vi "power calculations.vi"() -> ()   [LabVIEW 2012]
uses:
  <vilib>/measure/maspectr.llb/FFT Power Spectrum and PSD for 1 Chan.vi
  <instrlib>/niUSRP/niUSRP Fetch Rx Data (CDB Cluster).vi
  <vilib>/measure/NI_MAPro.lvlib
panel:
  in  "carrier frequency":dbl=100000.0 format="%#_6p"
  in  "gain":dbl format="%#_6f"
  in  "IQ rate":dbl=100000.0 format="%#_6p"
  out "x/y":dbl
  out "SNR":dbl
  out "Power Spectrum / PSD":cluster{"f0":dbl, "df":dbl, "magnitude":dbl[]} {"magnitude" format="%.2p"; "f0" format="%0.2p"; "df" format="%0.2p"}
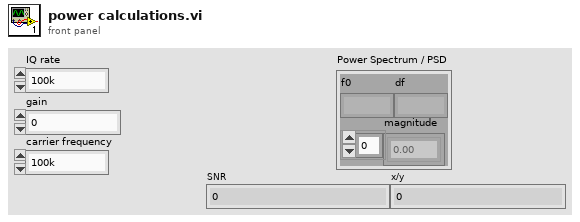
[diagram p1: front panel]
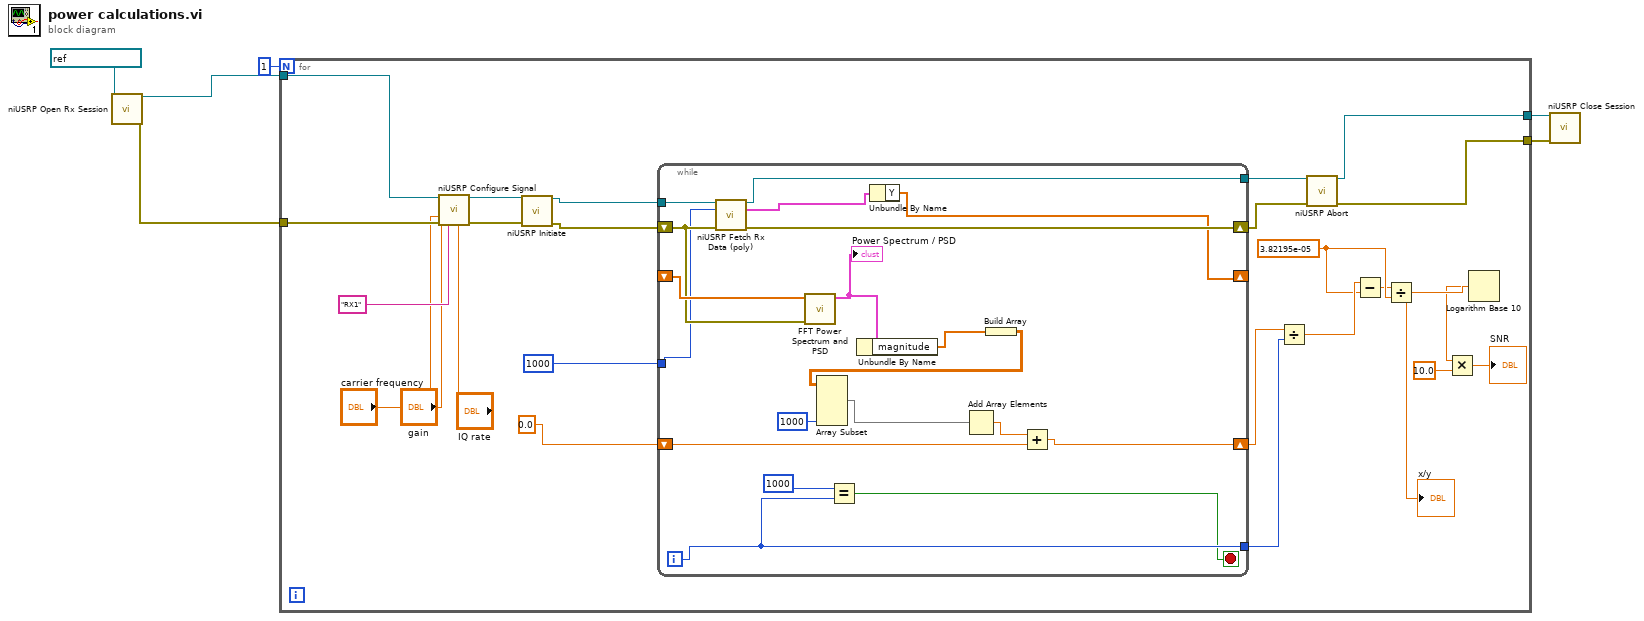
[diagram p0: block diagram]
diagram:
  n1 = call <instrlib>:"niUSRP Open Rx Session.vi"("device names"=refnum<k15> "192.168.10.4") -> ("session handle out"=w6:refnum<k15>, "error out"=w5:errorcluster)  [unwired: 13 in]
  n2 = for {
    N: 1 -> [_]
    tunnel: w6 -> [w31]
    tunnel: w5 -> [w28]
    tunnel: [w14] -> w2
    tunnel: [w13] -> w1
    w8 = 3.82195e-05 ("y")
    n3 = call <instrlib>:"niUSRP Configure Signal.vi"("session handle"=w31, "IQ rate"="IQ rate", "carrier frequency"="carrier frequency", "gain"="gain", "error in (no error)"=w28, "active antenna"="RX1") -> ("session handle out"=w30:refnum<k15>, "error out"=w29:errorcluster)  [unwired: 5 in, 3 out]
    n4 = call <instrlib>:"niUSRP Initiate.vi"("session handle"=w30, "error in (no error)"=w29) -> ("session handle out"=w27:refnum<k15>, "error out"=w26:errorcluster)  [unwired: 12 in]
    n5 = while {
      tunnel: w27 -> [w50]
      shift-right: [w34] -> w25
      shift-left: w26 -> [w47]
      tunnel: [w49] -> w24
      shift-right: [w32] -> _
      shift-left: _ -> [w48]
      shift-right: [w41] -> w22
      shift-left: 0.0 -> [w42]
      tunnel: [w36] -> w21
      tunnel: 1000 -> [w39]
      i -> [w36]
      stop <- w35 stop-if-true
      n6 = call-poly <instrlib>:"niUSRP Fetch Rx Data (poly).vi"("session handle"=w50, "number of samples"=w39, "error in (no error)"=w47) -> ("session handle out"=w49:refnum<k15>, "data"=w33:cluster{"t0":dbl, "dt":dbl, "Y":cdb[]}, "error out"=w34:errorcluster)  [unwired: 9 in, 1 out]
      n7 = call-poly <vilib>:"FFT Power Spectrum and PSD.vi"("error in (no error)"=w47, "time signal"=w48) -> ("Power Spectrum / PSD"=w46:cluster{"f0":dbl, "df":dbl, "magnitude":dbl[]})  [unwired: 6 in, 3 out]
      "Power Spectrum / PSD" <- w46
      n8 = Equal?(x=1000, y=w36) -> (x = y?=w35:bool)
      n9 = Unbundle By Name(w46) -> ("magnitude"=w45:dbl[])
      n10 = Unbundle By Name(w33) -> ("Y"=w32:cdb[])
      n11 = Build Array(w45) -> (w44:dbl[][])
      n12 = Array Subset(array=w44, length (col)=1000 ("length")) -> (w43:dbl[][])  [unwired: 3 in]
      n13 = Add Array Elements(numeric array=w43) -> (sum=w40:dbl)
      n14 = Add(x=w40, y=w42) -> (x+y=w41:dbl)
    }
    n15 = Divide(x=w22, y=w21) -> (x/y=w9:dbl)
    n16 = call <instrlib>:"niUSRP Abort.vi"("session handle"=w24, "error in (no error)"=w25) -> ("session handle out"=w14:refnum<k15>, "error out"=w13:errorcluster)  [unwired: 12 in]
    n17 = Subtract(x=w9, y=w8) -> (x-y=w7:dbl)
    n18 = Divide(x=w7, y=w8) -> (x/y=w20:dbl)
    "x/y" <- w20
    n19 = Logarithm Base 10(1:w20) -> (0:w19:dbl)
    n20 = Multiply(x=w19, y=10.0) -> (x*y=→"SNR":dbl)
  }
  n21 = call <instrlib>:"niUSRP Close Session.vi"("session handle"=w2, "error in (no error)"=w1) -> ()  [unwired: 13 in, 1 out]
